vi "main.vi"() -> ()   [LabVIEW 2010]
uses:
  common/xcontrols/XImage/XImage/XImage.xctl
  common/classes/ImageCollection/ImageCollection/ImageCollection.lvclass
  PositionSignals/PositionSignals.lvclass
panel:
  out "progress":u8(slide) scale=0.0..100.0
  in  "Line scan":refnum<class "ImageCollection.lvclass">(xcontrol)
  in  "index of first position channel":i32=2
  in  "number of position channels":i32=3
  in  "button:stop":bool
  in  "Reference stack":refnum<class "ImageCollection.lvclass">(xcontrol)
  # "Line Scan Analyzer"
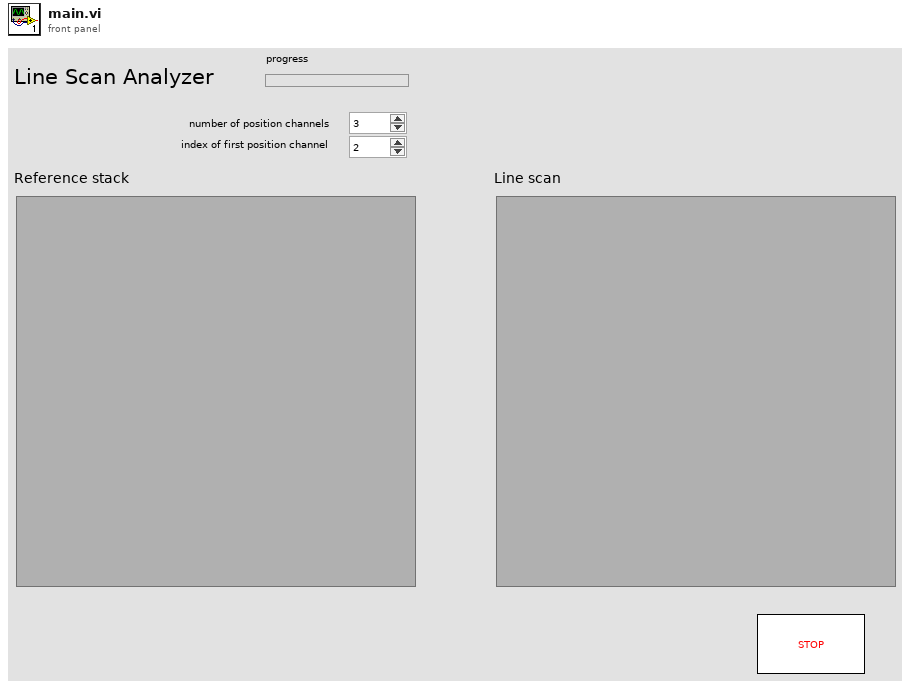
[diagram p1: front panel]
types:
  T1 = typedef "XImage.xctl/last_action_enum.ctl" = enum16{"not specified", "image loaded", "frame changed", "ROIs changed"}
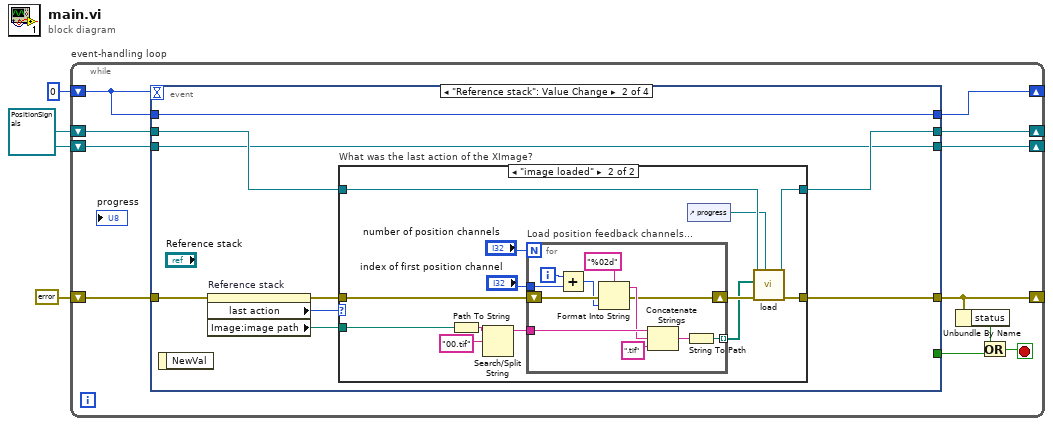
[diagram p0: block diagram]
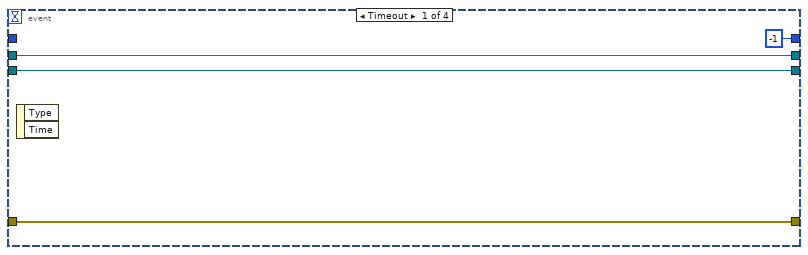
[diagram p2: hidden frame]
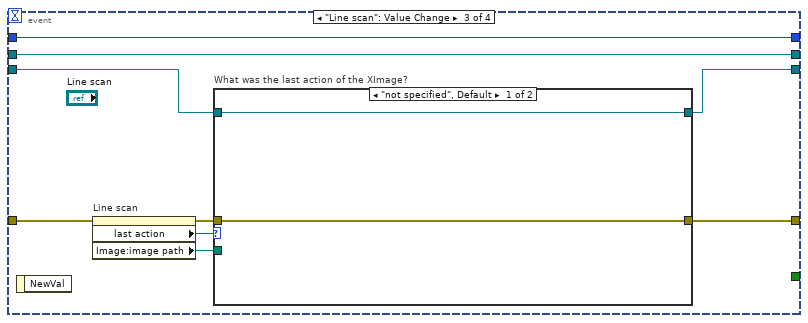
[diagram p4: hidden frame]
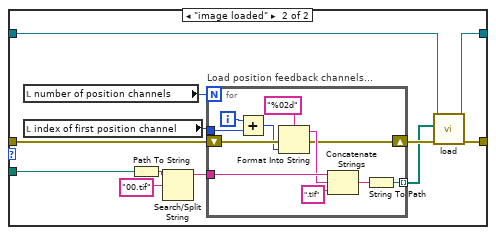
[diagram p5: hidden frame]
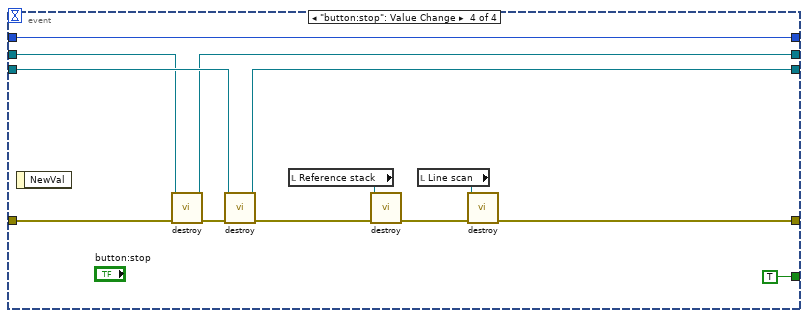
[diagram p6: hidden frame]
diagram:
  w1 = refnum<class "PositionSignals.lvclass"> refnum ("PositionSignals.lvclass")
  n1 = while "event-handling loop" {
    shift-right: [w13] -> _
    shift-left: errorcluster {"status"=FALSE, "code"=0, "source"=""} ("error in (no error)") -> [w14]
    shift-right: [w8] -> _
    shift-left: 0 -> [w9]
    shift-right: [w6] -> _
    shift-left: w1 -> [w7]
    shift-right: [w4] -> _
    shift-left: w1 -> [w5]
    stop <- w10 stop-if-true
    n2 = event shown="[1] \"Reference stack\": Value Change" {
      selector: _ -> [_ _ _ _]
      dyn-events: _ -> [_ _ _ _]
      timeout: w9 -> [_ _ _ _]
      tunnel: w14 -> [w15 w26 w57 w93]
      tunnel: [w15 w23 w54 w88] -> w13
      tunnel: [_ _ _ TRUE] -> w11
      tunnel: w9 -> [_ w27 w62 w99]
      tunnel: [-1 w27 w62 w99] -> w8
      tunnel: [w17 w21 w61 w96] -> w6
      tunnel: w7 -> [w17 w22 w61 w97]
      tunnel: w5 -> [w16 w19 w56 w98]
      tunnel: [w16 w19 w55 w95] -> w4
      event Timeout {
        n3 = event-data() -> ()  [unwired: 1 in, 2 out]
      }
      event "Reference stack": Value Change {
        n4 = event-data() -> ()  [unwired: 1 in, 1 out]
        n5 = property on="Reference stack" class="XImage (strict)"(error in=w26) -> (error out=w24:errorcluster, "last action"=w20:T1, "Image:image path"=w25:path)  [unwired: 1 in, 1 out]
        n6 = case "What was the last action of the XImage?" shown="\"image loaded\"" w20 {
          tunnel: w25 -> [_ w33]
          tunnel: w24 -> [w29 w36]
          tunnel: [w29 w42] -> w23
          tunnel: w22 -> [w28 w41]
          tunnel: [w28 w40] -> w21
          frame "not specified", Default {
          }
          frame "image loaded" {
            n7 = Path To String(path=w33) -> (string=w38:string)
            n8 = Search/Split String(string=w38, search string/char (-)="00.tif") -> (substring before match=w39:string)  [unwired: 1 in, 2 out]
            n9 = for "Load position feedback channels..." {
              N: "number of position channels" -> [_]
              shift-right: [w44] -> w35
              shift-left: w36 -> [w50]
              tunnel: w39 -> [w49]
              tunnel: "index of first position channel" -> [w45]
              tunnel: [w43] -> w34 mode=indexing
              i -> [w51]
              n10 = Add(x=w51, y=w45) -> (x+y=w46:i32)
              n11 = Format Into String(format string="%02d", error in=w50, w46) -> (resulting string=w48:string, error out=w44:errorcluster)  [unwired: 1 in]
              n12 = Concatenate Strings(w49, w48, ".tif" ("string")) -> (w53:string)
              n13 = String To Path(string=w53) -> (path=w43:path)
            }
            n14 = control-ref of="progress"() -> (w30:refnum<vi>)
            n15 = call "load.vi"("progress bar ref"=w30, "error in (no error)"=w35, "x/y/z path"=w34, "PositionSignals in"=w41) -> ("error out"=w42:errorcluster, "PositionSignals out"=w40:refnum<class "PositionSignals.lvclass">)  [unwired: 6 in]
          }
        }
      }
      event "Line scan": Value Change {
        n16 = event-data() -> ()  [unwired: 1 in, 1 out]
        n17 = property on="Line scan" class="XImage (strict)"(error in=w57) -> (error out=w59:errorcluster, "last action"=w58:T1, "Image:image path"=w60:path)  [unwired: 1 in, 1 out]
        n18 = case "What was the last action of the XImage?" shown="\"not specified\", Default" w58 {
          tunnel: w60 -> [_ w67]
          tunnel: w59 -> [w64 w70]
          tunnel: [w64 w76] -> w54
          tunnel: w56 -> [w63 w75]
          tunnel: [w63 w74] -> w55
          frame "not specified", Default {
          }
          frame "image loaded" {
            n19 = local read "number of position channels"() -> (w66:i32)
            n20 = local read "index of first position channel"() -> (w65:i32)
            n21 = Path To String(path=w67) -> (string=w72:string)
            n22 = Search/Split String(string=w72, search string/char (-)="00.tif") -> (substring before match=w73:string)  [unwired: 1 in, 2 out]
            n23 = for "Load position feedback channels..." {
              N: w66 -> [_]
              shift-right: [w78] -> w69
              shift-left: w70 -> [w84]
              tunnel: w73 -> [w83]
              tunnel: w65 -> [w79]
              tunnel: [w77] -> w68 mode=indexing
              i -> [w85]
              n24 = Add(x=w85, y=w79) -> (x+y=w80:i32)
              n25 = Format Into String(format string="%02d", error in=w84, w80) -> (resulting string=w82:string, error out=w78:errorcluster)  [unwired: 1 in]
              n26 = Concatenate Strings(w83, w82, ".tif" ("string")) -> (w87:string)
              n27 = String To Path(string=w87) -> (path=w77:path)
            }
            n28 = call "load.vi"("error in (no error)"=w69, "x/y/z path"=w68, "PositionSignals in"=w75) -> ("error out"=w76:errorcluster, "PositionSignals out"=w74:refnum<class "PositionSignals.lvclass">)  [unwired: 7 in]
          }
        }
      }
      event "button:stop": Value Change {
        n29 = event-data() -> ()  [unwired: 1 in, 1 out]
        n30 = call "destroy.vi"("error in (no error)"=w93, "PositionSignals in"=w97) -> ("error out"=w94:errorcluster, "PositionSignals out"=w96:refnum<class "PositionSignals.lvclass">)  [unwired: 8 in]
        n31 = call "destroy.vi"("error in (no error)"=w94, "PositionSignals in"=w98) -> ("error out"=w89:errorcluster, "PositionSignals out"=w95:refnum<class "PositionSignals.lvclass">)  [unwired: 8 in]
        n32 = local read "Reference stack"() -> (w92:refnum<class "ImageCollection.lvclass">)
        n33 = call-dynamic "destroy.vi"("error in (no error)"=w89, "ImageCollection in"=w92) -> ("error out"=w90:errorcluster)  [unwired: 8 in, 1 out]
        n34 = local read "Line scan"() -> (w91:refnum<class "ImageCollection.lvclass">)
        n35 = call-dynamic "destroy.vi"("error in (no error)"=w90, "ImageCollection in"=w91) -> ("error out"=w88:errorcluster)  [unwired: 8 in, 1 out]
      }
    }
    n36 = Unbundle By Name(w13) -> ("status"=w12:bool)
    n37 = Or(x=w12, y=w11) -> (x .or. y?=w10:bool)
  }
